vi "DataVIS_Configure_Intensity_Plot.vi"(7 "Scan Name":string, 8 "error in (no error)":errorcluster, 9 "Y Offset and Multiplier":T1, 10 "X Offset and Multiplier":T1, 11 "IntensityGraph in":refnum<vi>) -> (0 "error out":errorcluster)   [LabVIEW 2016]
uses:
  <vilib>/Utility/miscctls.llb/LVOffsetAndMultiplierTypeDef.ctl
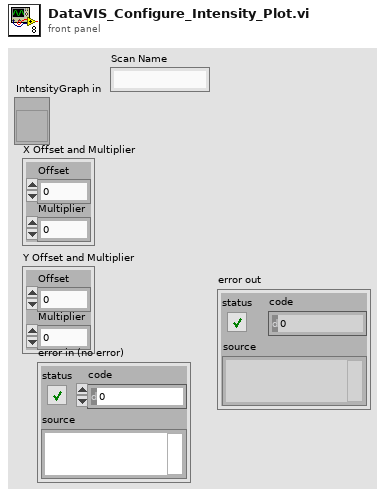
[diagram p1: front panel]
types:
  T1 = typedef "LVOffsetAndMultiplierTypeDef.ctl" = cluster{"Offset":dbl, "Multiplier":dbl}
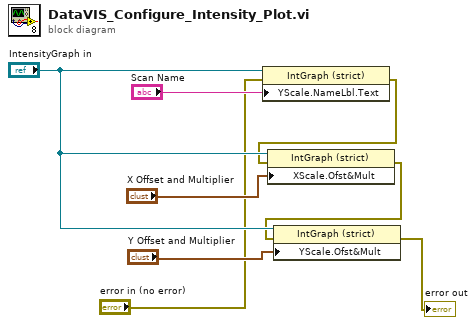
[diagram p0: block diagram]
diagram:
  n1 = property class="IntGraph (strict)"(reference="IntensityGraph in", error in="error in (no error)", "YScale.NameLbl.Text"="Scan Name") -> (error out=w2:errorcluster)  [unwired: 1 out]
  n2 = property class="IntGraph (strict)"(reference="IntensityGraph in", error in=w2, "XScale.Ofst&Mult"="X Offset and Multiplier") -> (error out=w3:errorcluster)  [unwired: 1 out]
  n3 = property class="IntGraph (strict)"(reference="IntensityGraph in", error in=w3, "YScale.Ofst&Mult"="Y Offset and Multiplier") -> (error out=→"error out":errorcluster)  [unwired: 1 out]
